vi "Enable Resistance Measurement.vi"(0 "VISA resource name":refnum<visa-resource-name>, 1 "Enable Resistance Measurement (F: Disable)":bool, 11 "error in (no error)":errorcluster) -> (4 "VISA resource name out":refnum<visa-resource-name>, 15 "error out":errorcluster)   [LabVIEW 2021, in "Keithley 648X Series.lvlib"]
doc: "Enables or disables the ohms function. When this function is enabled the instrument calculates the reading from the measured current and voltage setting using the equation R = V/I.\n\n<b>Note:</b>\nThis VI supports Model 6487 only"
uses:
  <instrlib>/Keithley 648X Series/Keithley 648X Series.lvlib
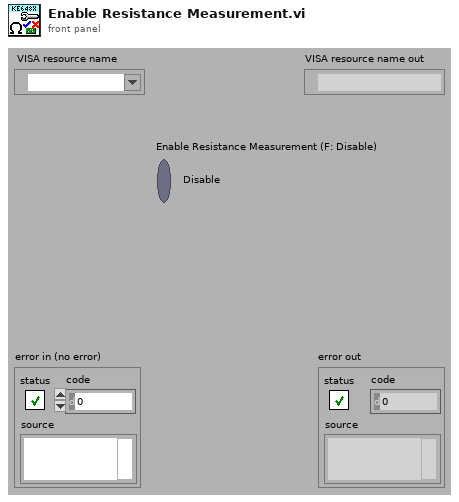
[diagram p1: front panel]
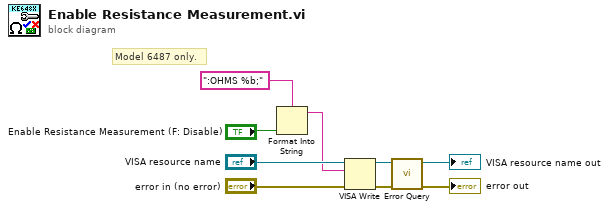
[diagram p0: block diagram]
diagram:
  # "Model 6487 only."
  n1 = Format Into String(format string=":OHMS %b;", "Enable Resistance Measurement (F: Disable)") -> (resulting string=w1:string)  [unwired: 2 in, 1 out]
  n2 = VISA Write(VISA resource name="VISA resource name", write buffer=w1, error in (no error)="error in (no error)") -> (VISA resource name out=w5:refnum<visa-resource-name>, error out=w4:errorcluster)  [unwired: 1 out]
  n3 = call <instrlib>:"Error Query.vi"("error in (no error)"=w4, "VISA resource name"=w5) -> ("error out"=→"error out":errorcluster, "VISA resource name out"=→"VISA resource name out":refnum<visa-resource-name>)  [unwired: 6 in, 2 out]
